vi "Go At Angle.vi"(0 "Target Angle":dbl, 2 "Bot Angle":dbl=6.265957027809849, 3 "dt":dbl=0.03, 5 "Stop motors":bool, 6 "Speed":T1={"\nMoving speed"=1.0296610169491527, "Turning speed limit"=1.0169491525423728} {"Turning speed limit" scale=0.0..4.5; "Moving speed" scale=0.0..1.0}) -> ()   [LabVIEW 2017]
uses:
  <vilib>/addons/control/pid/pid.llb/PID (DBL).vi
  Globals/Motor Speed Multiplier.vi
  <vilib>/addons/control/pid/NI_PID_pid.lvlib
panel:
  in  "Turning PID":cluster{"P":dbl, "I":dbl, "D":dbl}={"P"=-0.8, "I"=0.0, "D"=0.007}
  in  "threshold angle":dbl=0.3
  out "Right motor speed":dbl=0.013786667806161291
  out "Left motor speed":dbl=-0.013786667806161291
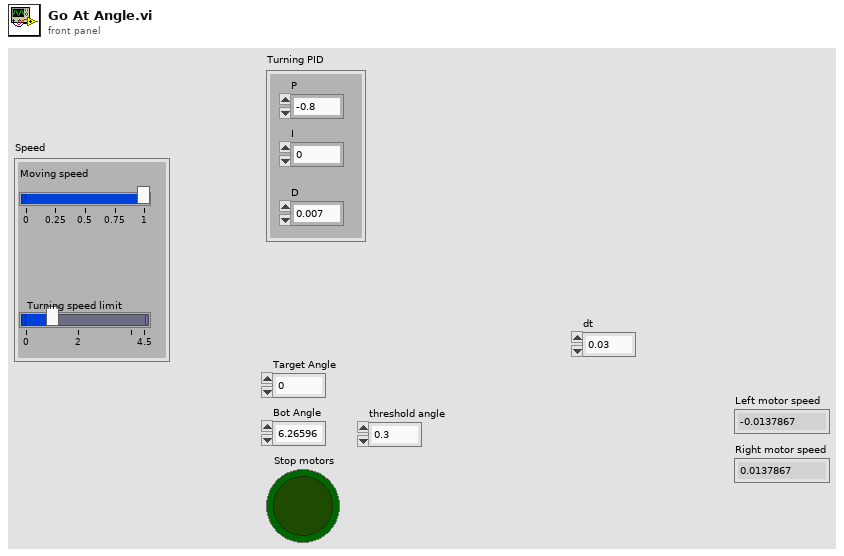
[diagram p1: front panel]
types:
  T1 = cluster{"\nMoving speed":dbl, "Turning speed limit":dbl}
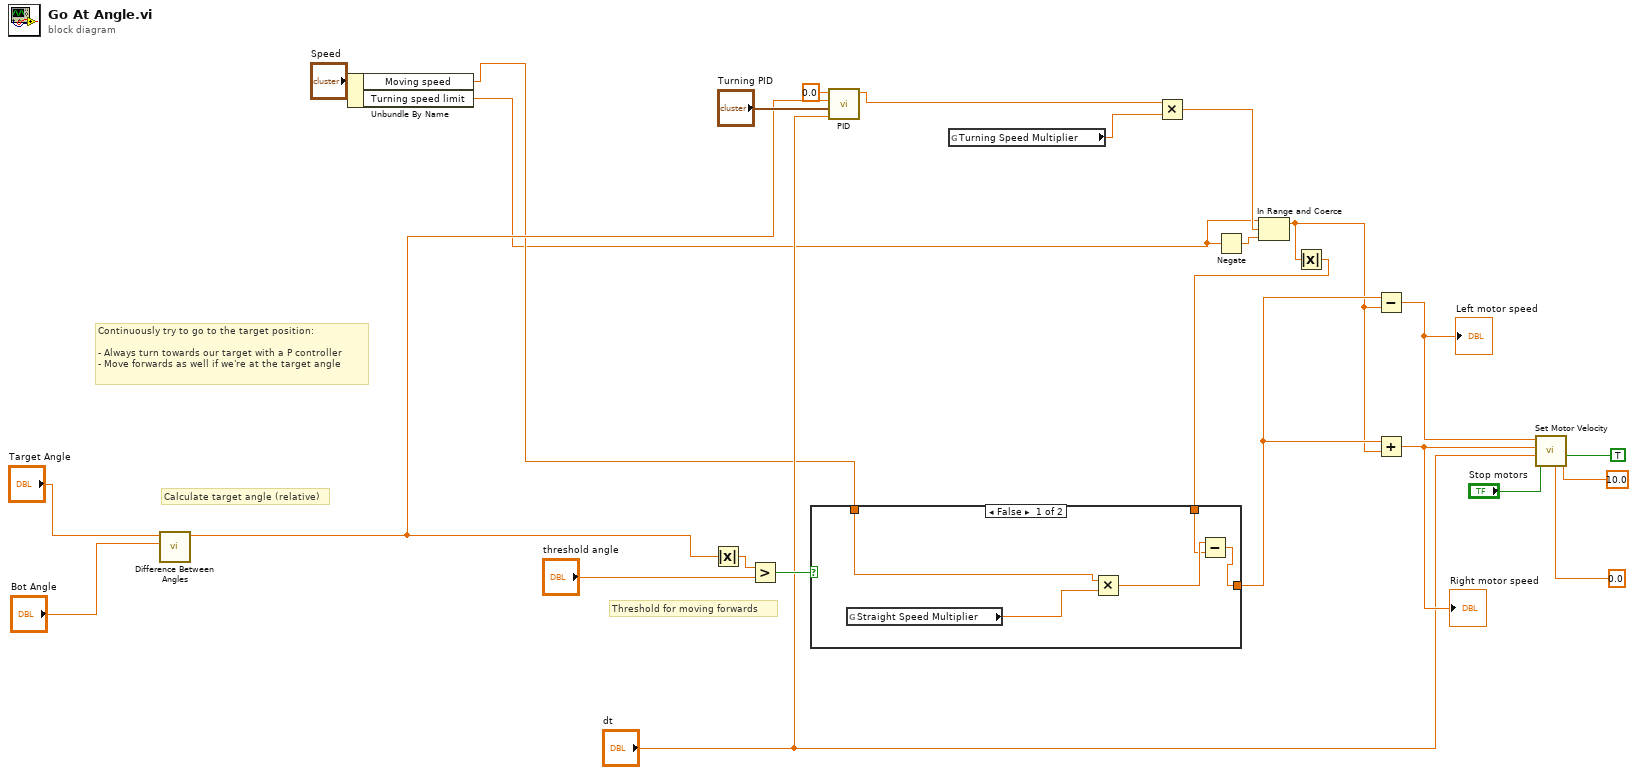
[diagram p0: block diagram]
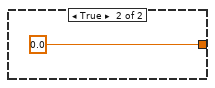
[diagram p2: hidden frame]
diagram:
  # "Threshold for moving forwards"
  # "Calculate target angle (relative)"
  # "Continuously try to go to the target position:\n\n- Always turn towards our target with a P controller\n- Move forwards as well if we're at the target angle"
  n1 = call "Difference Between Angles.vi"("Angle 2"="Bot Angle", "Angle 1"="Target Angle") -> ("Difference"=w8:dbl)  [unwired: 9 in]
  n2 = Unbundle By Name("Speed") -> ("Moving speed"=w5:dbl, "Turning speed limit"=w4:dbl)
  n3 = Absolute Value(x=w8) -> (abs(x)=w20:dbl)
  n4 = Greater?(x=w20, y="threshold angle") -> (0:w16:bool)
  n5 = call-poly <vilib>:"PID.vi"("dt (s)"="dt", "PID gains"="Turning PID", "process variable"=w8, "setpoint"=0.0) -> ("output"=w3:dbl)  [unwired: 6 in, 1 out]
  n6 = global read "Motor Speed Multiplier.vi" "Turning Speed Multiplier"() -> (w2:dbl)
  n7 = Multiply(x=w3, y=w2) -> (x*y=w14:dbl)
  n8 = Negate(x=w4) -> (-x=w13:dbl)
  n9 = In Range and Coerce(upper limit=w4, x=w14, lower limit=w13) -> (coerced(x)=w12:dbl)  [unwired: 1 out]
  n10 = Absolute Value(x=w12) -> (abs(x)=w11:dbl)
  n11 = case shown="False" w16 {
    tunnel: [w27 0.0] -> w17
    tunnel: w11 -> [w28 _]
    tunnel: w5 -> [w26 _]
    frame False {
      n12 = global read "Motor Speed Multiplier.vi" "Straight Speed Multiplier"() -> (w30:dbl)
      n13 = Multiply(x=w26, y=w30) -> (x*y=w29:dbl)
      n14 = Subtract(x=w29, y=w28) -> (x-y=w27:dbl)
    }
    frame True {
    }
  }
  n15 = Subtract(x=w17, y=w12) -> (x-y=w18:dbl)
  "Left motor speed" <- w18
  n16 = Add(x=w17, y=w12) -> (x+y=w19:dbl)
  "Right motor speed" <- w19
  n17 = call "Set Motor Velocity.vi"("Acceleration ramp constant"=10.0, "Accelerate?"=TRUE, "Back motor speed rev/s"=0.0 ("result"), "Disable motors"="Stop motors", "dt"="dt", "Right motor speed rev/s"=w19, "Left motor speed rev/s"=w18) -> ()  [unwired: 5 in]
